vi "Comm String Send Script.vi"(0 "niDTS Comm String in":refnum<class "niDTS Comm String.lvclass">, 5 "script":string, 11 "error in (no error)":errorcluster) -> (4 "niDTS Comm String out":refnum<class "niDTS Comm String.lvclass">, 6 "Return":string, 15 "error out":errorcluster)   [LabVIEW 2015, in "niDTS CommLib.lvlib" / "niDTS Comm String.lvclass"]
uses:
  niDTS Comm String.lvclass
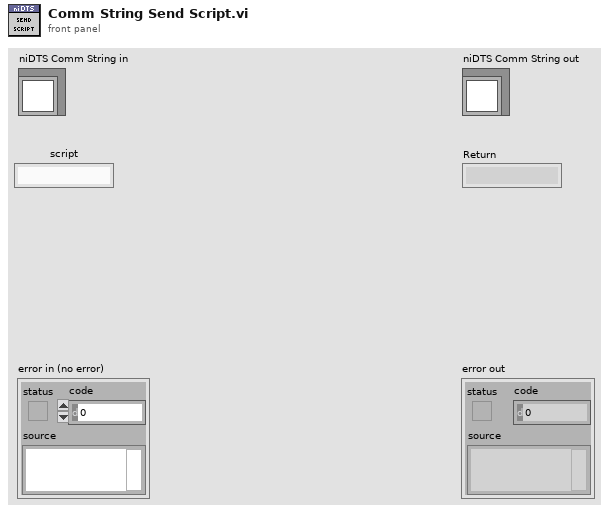
[diagram p1: front panel]
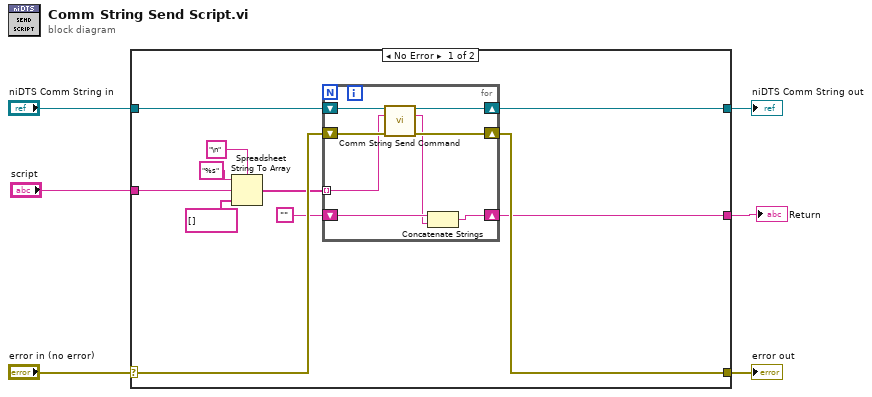
[diagram p0: block diagram]
diagram:
  n1 = case shown="No Error" "error in (no error)" {
    selector: "error in (no error)" -> [w11 w27]
    tunnel: [w10 w27] -> w5
    tunnel: [w12 w26] -> w3
    tunnel: "niDTS Comm String in" -> [w13 w26]
    tunnel: "script" -> [w14 _]
    tunnel: [w7 _] -> w1
    frame No Error {
      n2 = Spreadsheet String To Array(delimiter (Tab)="\n", format string="%s", spreadsheet string=w14, array type (2D Dbl)=string[] []) -> (array=w9:string[])
      n3 = for {
        shift-right: [w24] -> w12
        shift-left: w13 -> [w25]
        shift-right: [w23] -> w10
        shift-left: w11 -> [w22]
        tunnel: w9 -> [w21] mode=indexing
        shift-right: [w18] -> w7
        shift-left: "" -> [w20]
        n4 = call-dynamic "Comm String Send Command.vi"("niDTS Comm String in"=w25, "Command"=w21, "error in (no error)"=w22) -> ("niDTS Comm String out"=w24:refnum<class "niDTS Comm String.lvclass">, "Response"=w19:string, "error out"=w23:errorcluster)  [unwired: 10 in]
        n5 = Concatenate Strings(w20, w19) -> (w18:string)
      }
    }
    frame Error {
    }
  }
  "error out" <- w5
  "niDTS Comm String out" <- w3
  "Return" <- w1
